vi "save_results.vi"() -> ()   [LabVIEW 2013]
uses:
  <vilib>/addons/database/Connection.llb/DB Tools Open Connec (String).vi
  <vilib>/addons/database/Connection.llb/Conn Execute.vi
  <vilib>/addons/database/Recordset.llb/Rec Fetch Recordset Data (R).vi
  <vilib>/addons/database/Recordset.llb/Rec Destroy - Connection.vi
  <vilib>/addons/database/NI_Database_API.lvlib
  FT_HMI.llb/GLOBAL_PUMPS_PARAMS.vi
  FT_HMI.llb/GLOBAL_GEN.vi
  FT_HMI.llb/GLOBAL_RESULT.vi
  <vilib>/addons/database/Connection.llb/Conn Get Properties.vi
  <vilib>/addons/database/Recordset.llb/Rec Fetch Integer Data (R).vi
  ADS.llb/Global DIOs.vi
panel:
  out "recordset data":variant[][](array[variant])
  out "subarray":variant[](array[variant])
  in  "SAVE":bool
  in  "Cluster 2":T1
  out "Nbre de lignes 4":i32
  in  "stop":bool
  in  "no article":string
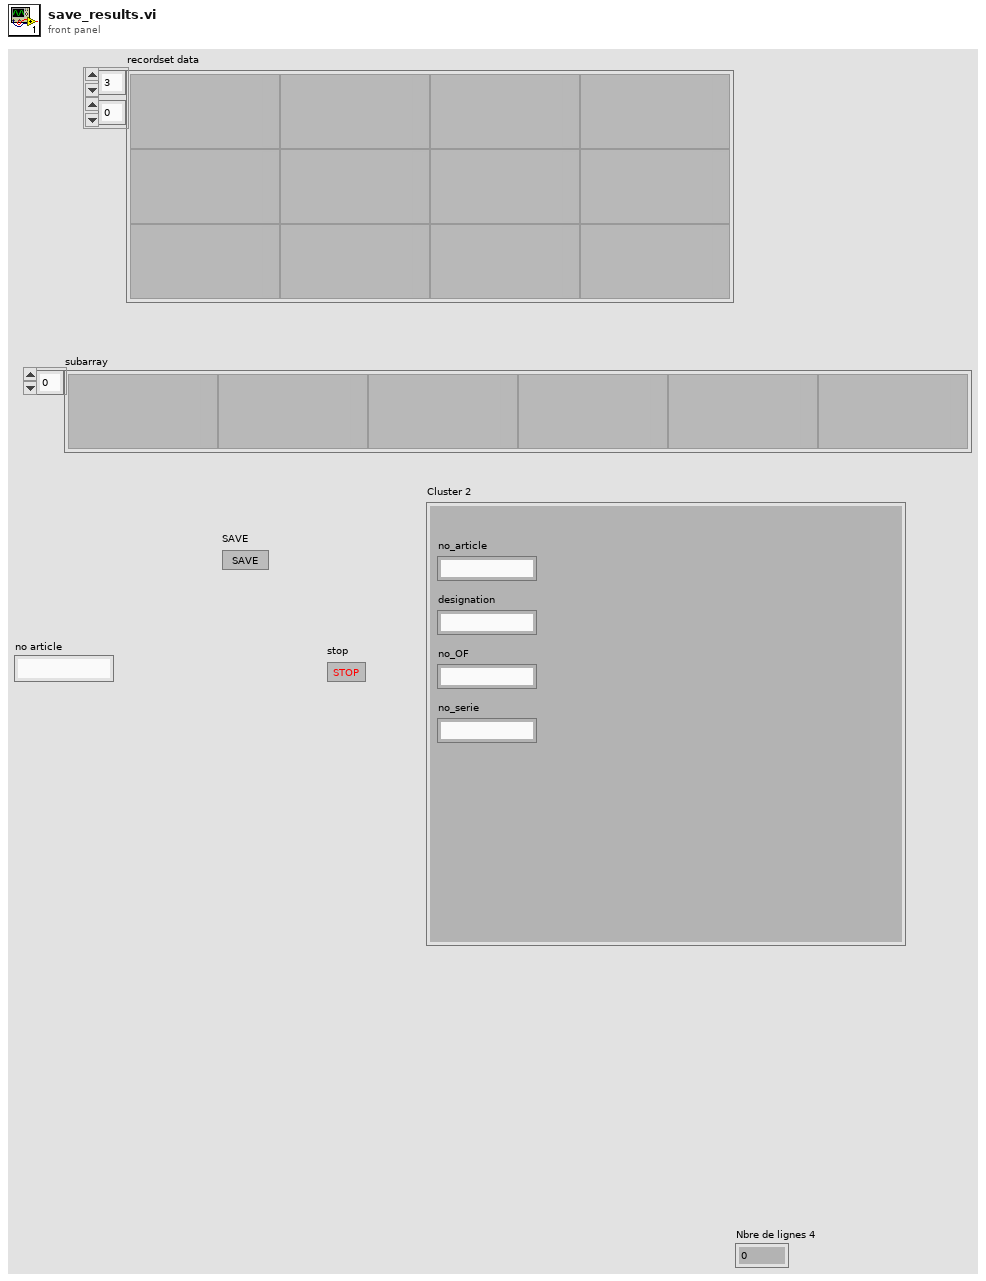
[diagram p1: front panel]
types:
  T1 = cluster{"no_article":string, "designation":string, "no_OF":string, "no_serie":string}
  T2 = typedef "NI_Database_API.lvlib/Conn ObjectReference.ctl" = refnum<k1>
  T3 = typedef "NI_Database_API.lvlib/Rec ObjectReference.ctl" = refnum<k1>
  T4 = cluster{"GENERAL":cluster{"NO_ARTICLE":string, "DESIGNATION":string}, "ALIMENTATION":cluster{"VOLTAGE [V]":sgl, "FREQUENCY [Hz]":sgl}, "ST1_HT":cluster{"ENABLE":bool, "TENSION ISOLATION [V]":sgl, "COURANT ISOLATION [mA]":sgl, "TEMPS DE MESURE [s]":sgl, "NO PROGRAMME":i32}, "ST2_ASPIRATION":cluster{"ENABLE_H_ASP":bool, "HAUTEUR ASPIRATION [m]":sgl, "TEMPS DE MESURE ASP [s]":sgl, "ENABLE_PERTE_ASP":bool, "PERTE ASPIRATION [mbar]":sgl, "TEMPS DE MESURE PERTE [s] ":sgl}, "ST3_ETANCHEITE":cluster{"ENABLE":bool, "ETANCHEITE [mbar]":sgl, "TEMPS DE MESURE [s]":sgl}, "ST4-5_DEBIT":cluster{"ENABLE_QMAX":bool, "TYPE DEBIT":i8, "PUMPING_TIME  [ms]":sgl, "DEBIT MIN [l/h]":sgl, "DEBIT MAX  [l/h]":sgl, "TEMPS DE MESURE QMAX [s]":sgl, "ENABLE_QTRAVAIL":bool, "DEBIT TRAVAIL [l/h]":sgl, "PRESSION DE CONSIGNE [bar]":sgl, "TEMPS DE MESURE QTRAVAIL [s]":sgl, "ENABLE_CONSO":bool, "CONSOMMATION [A]":sgl, "TEMPS DE MESURE COURANT [s]":sgl}, "ST6_PRESSION":cluster{"ENABLE_PMAX":bool, "PUMPING_TIME [ms]":sgl, "PRESSION MIN [bar]":sgl, "TEMPS DE MESURE PMAX [s]":sgl, "ENABLE_PERTE_PRESSION":bool, "PERTE PRESSION [mbar]":sgl, "TEMPS DE MESURE PERTE [s]":sgl}, "ST7_VIDANGE":cluster{"ENABLE":bool, "TEMPS DE VIDANGE [S] ":sgl}, "ST8_IMPRESSION":cluster{"ENABLE":bool}, "ST9_DECHARGEMENT":cluster{"ENABLE":bool}}
  T5 = typedef "TYPE_DEF_PUMP_RESULTS.ctl" = cluster{"Test HT":i16, "Aspiration [m]":sgl, "Perte asp [mbar]":sgl, "Etancheite [mbar]":sgl, "Debit max [l/h]":sgl, "Débit travail [l/h]":sgl, "Courant max [mA]":sgl, "By-pass":i16, "Pression max [bar]":sgl, "Perte pression [mbar]":sgl, "Pump status":bool}
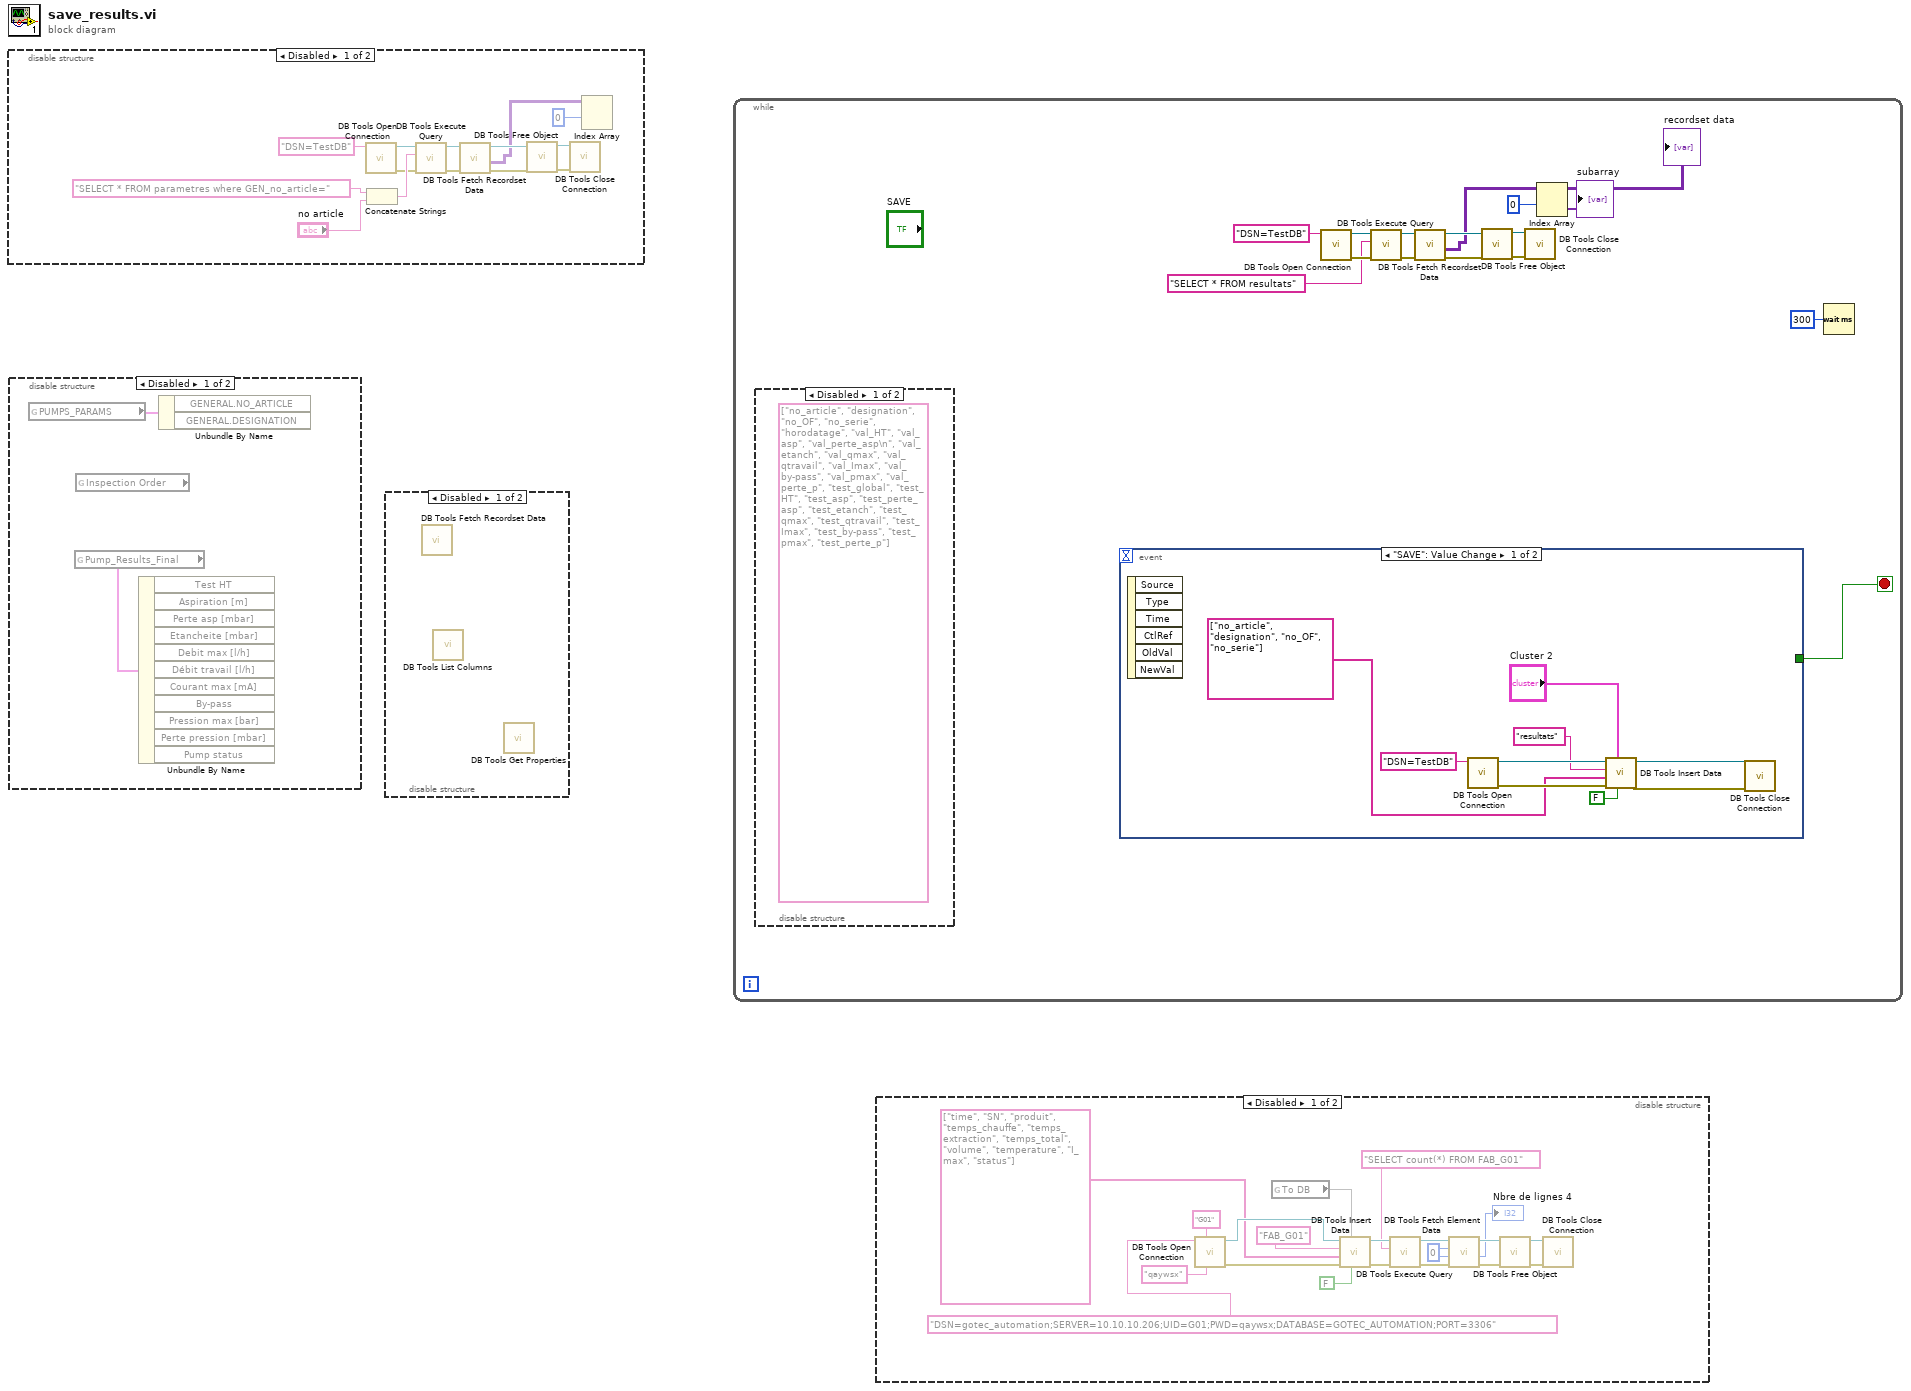
[diagram p0: block diagram]
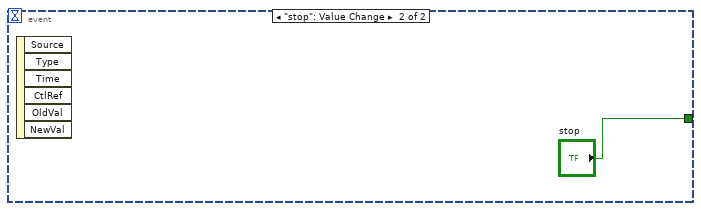
[diagram p3: hidden frame]
diagram:
  n1 = disable-structure shown="Disabled" {
    frame Disabled {
      n2 = call-poly <vilib>:"DB Tools Open Connection.vi"("connection information"="DSN=TestDB") -> ("error out"=w4:errorcluster, "connection reference"=w5:T2)  [unwired: 7 in]
      n3 = Concatenate Strings("SELECT * FROM parametres where GEN_no_article=" ("SQL query"), "no article") -> (w7:string)
      n4 = call-poly <vilib>:"DB Tools Execute Query.vi"("error in (no error)"=w4, "SQL query"=w7, "connection reference"=w5) -> ("error out"=w10:errorcluster, "recordset reference"=w12:T3)  [unwired: 5 in]
      n5 = call-poly <vilib>:"DB Tools Fetch Recordset Data.vi"("error in (no error)"=w10, "recordset reference"=w12) -> ("error out"=w9:errorcluster, "recordset data"=w1:variant[][], "recordset reference out"=w11:T3)  [unwired: 3 in]
      n6 = call-poly <vilib>:"DB Tools Free Object.vi"("error in (no error)"=w9, "recordset reference"=w11) -> ("error out"=w13:errorcluster, "connection reference"=w2:T2)  [unwired: 8 in]
      n7 = call <vilib>:"DB Tools Close Connection.vi"("error in (no error)"=w13, "connection reference"=w2) -> ()  [unwired: 5 in, 1 out]
      n8 = Index Array(array=w1, index (row)=0 ("index")) -> ()  [unwired: 1 in, 1 out]
    }
    frame Enabled {
    }
  }
  n9 = disable-structure shown="Disabled" {
    frame Disabled {
      n10 = global read "GLOBAL_PUMPS_PARAMS.vi" "PUMPS_PARAMS"() -> (w16:T4)
      n11 = global read "GLOBAL_RESULT.vi" "Pump_Results_Final"() -> (w15:T5)
      n12 = global read "GLOBAL_GEN.vi" "Inspection Order"() -> ()  [unwired: 1 out]
      n13 = Unbundle By Name(w15) -> ()  [unwired: 11 out]
      n14 = Unbundle By Name(w16) -> ()  [unwired: 2 out]
    }
    frame Enabled {
    }
  }
  n15 = disable-structure shown="Disabled" {
    frame Disabled {
      n16 = call-poly <vilib>:"DB Tools Fetch Recordset Data.vi"() -> ()  [unwired: 5 in, 3 out]
      n17 = call <vilib>:"DB Tools List Columns.vi"() -> ()  [unwired: 4 in, 4 out]
      n18 = call-poly <vilib>:"DB Tools Get Properties.vi"() -> ()  [unwired: 5 in, 3 out]
    }
    frame Enabled {
    }
  }
  n19 = while {
    stop <- w30 stop-if-true
    n20 = disable-structure shown="Disabled" {
      frame Disabled {
        w42 = string[] ["no_article", "designation", "no_OF", "no_serie", "horodatage", "val_HT", "val_asp", "val_perte_asp\n", "val_etanch", "val_qmax", "val_qtravail", "val_Imax", "val_by-pass", "val_pmax", "val_perte_p", "test_global", "test_HT", "test_asp", "test_perte_asp", "test_etanch", "test_qmax", "test_qtravail", "test_Imax", "test_by-pass", "test_pmax", "test_perte_p"] ("columns")
      }
      frame Enabled {
      }
    }
    n21 = event shown="[0] \"SAVE\": Value Change" {
      selector: _ -> [_ _]
      dyn-events: _ -> [_ _]
      timeout: _ -> [_ _]
      tunnel: [_ "stop"] -> w30
      event "SAVE": Value Change {
        n22 = event-data() -> ()  [unwired: 1 in, 6 out]
        n23 = call-poly <vilib>:"DB Tools Open Connection.vi"("connection information"="DSN=TestDB") -> ("error out"=w37:errorcluster, "connection reference"=w38:T2)  [unwired: 7 in]
        n24 = call <vilib>:"DB Tools Insert Data.vi"("flatten cluster? (F)"=FALSE ("use file? (F)"), "data"="Cluster 2", "error in (no error)"=w37, "columns"=string[] ["no_article", "designation", "no_OF", "no_serie"], "table"="resultats", "connection reference"=w38) -> ("error out"=w35:errorcluster, "connection reference out"=w36:T2)  [unwired: 4 in]
        n25 = call <vilib>:"DB Tools Close Connection.vi"("error in (no error)"=w35, "connection reference"=w36) -> ()  [unwired: 5 in, 1 out]
      }
      event "stop": Value Change {
        n26 = event-data() -> ()  [unwired: 1 in, 6 out]
      }
    }
    n27 = call-poly <vilib>:"DB Tools Open Connection.vi"("connection information"="DSN=TestDB") -> ("error out"=w22:errorcluster, "connection reference"=w23:T2)  [unwired: 7 in]
    n28 = call-poly <vilib>:"DB Tools Execute Query.vi"("error in (no error)"=w22, "SQL query"="SELECT * FROM resultats", "connection reference"=w23) -> ("error out"=w25:errorcluster, "recordset reference"=w27:T3)  [unwired: 5 in]
    n29 = call-poly <vilib>:"DB Tools Fetch Recordset Data.vi"("error in (no error)"=w25, "recordset reference"=w27) -> ("error out"=w24:errorcluster, "recordset data"=w19:variant[][], "recordset reference out"=w26:T3)  [unwired: 3 in]
    "recordset data" <- w19
    n30 = call-poly <vilib>:"DB Tools Free Object.vi"("error in (no error)"=w24, "recordset reference"=w26) -> ("error out"=w28:errorcluster, "connection reference"=w20:T2)  [unwired: 8 in]
    n31 = call <vilib>:"DB Tools Close Connection.vi"("error in (no error)"=w28, "connection reference"=w20) -> ()  [unwired: 5 in, 1 out]
    n32 = Index Array(array=w19, index (row)=0 ("index")) -> (element=→"subarray":variant[])  [unwired: 1 in]
    n33 = Wait (ms)(milliseconds to wait=u32 300) -> ()  [unwired: 1 out]
  }
  n34 = disable-structure shown="Disabled" {
    frame Disabled {
      w47 = 0
      n35 = call-poly <vilib>:"DB Tools Open Connection.vi"("password"="qaywsx", "userID"="G01", "connection information"="DSN=gotec_automation;SERVER=10.10.10.206;UID=G01;PWD=qaywsx;DATABASE=GOTEC_AUTOMATION;PORT=3306") -> ("error out"=w59:errorcluster, "connection reference"=w60:T2)  [unwired: 5 in]
      n36 = global read "Global DIOs.vi" "To DB"() -> (w43)
      n37 = call <vilib>:"DB Tools Insert Data.vi"("flatten cluster? (F)"=FALSE, "data"=w43, "error in (no error)"=w59, "columns"=string[] ["time", "SN", "produit", "temps_chauffe", "temps_extraction", "temps_total", "volume", "temperature", "I_max", "status"], "table"="FAB_G01", "connection reference"=w60) -> ("error out"=w50:errorcluster, "connection reference out"=w51:T2)  [unwired: 4 in]
      n38 = call-poly <vilib>:"DB Tools Execute Query.vi"("error in (no error)"=w50, "SQL query"="SELECT count(*) FROM FAB_G01", "connection reference"=w51) -> ("error out"=w56:errorcluster, "recordset reference"=w52:T3)  [unwired: 5 in]
      n39 = call-poly <vilib>:"DB Tools Fetch Element Data.vi"("error in (no error)"=w56, "type"=w47, "column index"=w47, "recordset reference"=w52) -> ("error out"=w55:errorcluster, "data"=→"Nbre de lignes 4":i32, "recordset reference out"=w53:T3)  [unwired: 3 in]
      n40 = call-poly <vilib>:"DB Tools Free Object.vi"("error in (no error)"=w55, "recordset reference"=w53) -> ("error out"=w49:errorcluster, "connection reference"=w54:T2)  [unwired: 8 in]
      n41 = call <vilib>:"DB Tools Close Connection.vi"("error in (no error)"=w49, "connection reference"=w54) -> ()  [unwired: 5 in, 1 out]
    }
    frame Enabled {
    }
  }
